vi "WalkOnAssertions.vi"(6 "Stop on 1st fail":bool, 7 "Banana":refnum<class "Banana.lvclass">, 8 "error in (no error)":errorcluster, 10 "Properties":refnum<class "Properties.Assert.lvclass">) -> (0 "error out":errorcluster, 2 "Properties out":refnum<class "Properties.Assert.lvclass">)   [LabVIEW 2021, in "Bananas.lvlib" / "Platano.lvclass"]
uses:
  Platano/Platano.lvclass
  BananaPeel/BananaPeel.lvclass
  Banana.lvclass
  <vilib>/addons/_JKI Toolkits/Caraya/classes/Properties.Assert/Properties.Assert.lvclass
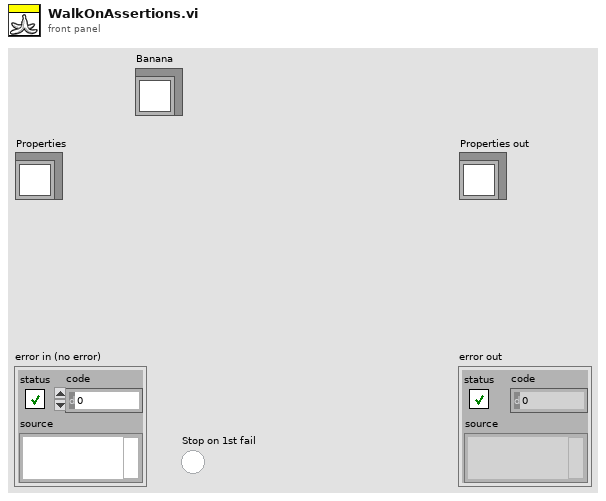
[diagram p1: front panel]
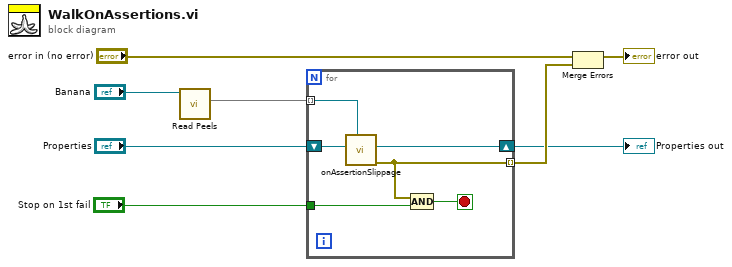
[diagram p0: block diagram]
diagram:
  n1 = call "Read Peels.vi"("Banana in"="Banana") -> ("Peels"=w1:set{refnum<class "BananaPeel.lvclass">})  [unwired: 8 in, 2 out]
  n2 = for {
    tunnel: [w11] -> w8 mode=indexing
    shift-right: [w13] -> w5
    shift-left: "Properties" -> [w14]
    tunnel: w1 -> [w12] mode=indexing
    tunnel: "Stop on 1st fail" -> [w10]
    stop <- w9 stop-if-true
    n3 = call-dynamic "onAssertionSlippage.vi"("BananaPeel in"=w12, "Properties"=w14) -> ("error out"=w11:errorcluster, "Properties out"=w13:refnum<class "Properties.Assert.lvclass">)  [unwired: 8 in]
    n4 = Compound Arithmetic op=AND(w11, w10) -> (w9:bool)
  }
  "Properties out" <- w5
  n5 = Merge Errors("error in (no error)", w8) -> (→"error out":errorcluster)
